vi "Decode Status.vi"(8 "error in (no error)":errorcluster, 10 "Status Line":string) -> (0 "error out":errorcluster, 1 "Checksum OK":bool, 2 "Output":i32)   [LabVIEW 2016]
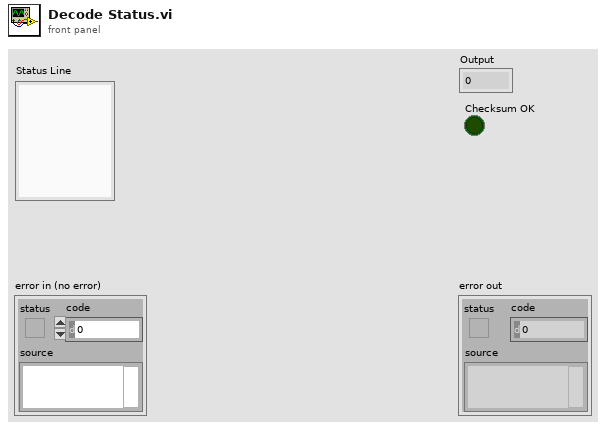
[diagram p1: front panel]
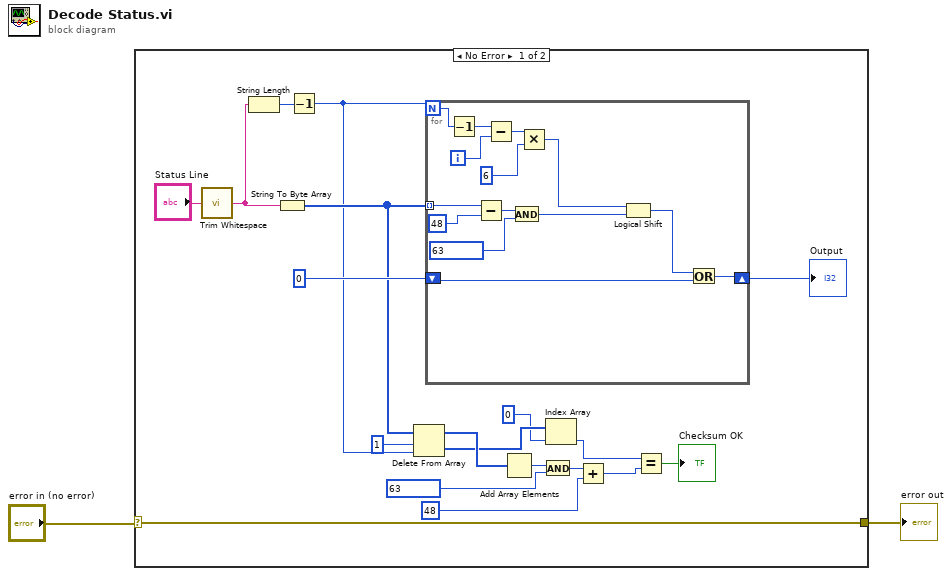
[diagram p0: block diagram]
diagram:
  n1 = case shown="No Error" "error in (no error)" {
    selector: "error in (no error)" -> [w3 w36]
    tunnel: [w3 w36] -> w1
    frame No Error {
      n2 = call <vilib>:"Trim Whitespace.vi"("string"="Status Line") -> ("trimmed string"=w4:string)  [unwired: 1 in]
      n3 = String Length(string=w4) -> (length=w21:i32)
      n4 = String To Byte Array(string=w4) -> (unsigned byte array=w12:u8[])
      n5 = Decrement(x=w21) -> (x-1=w7:i32)
      n6 = Delete From Array(array=w12, length=1, index=w7) -> (deleted portion=w11:u8[], array with subset deleted=w14:u8[])
      n7 = for {
        N: w7 -> [w26]
        tunnel: w12 -> [w22] mode=indexing
        shift-right: [w34] -> w20
        shift-left: 0 -> [w33]
        i -> [w31]
        n8 = Decrement(x=w26) -> (x-1=w25:i32)
        n9 = Subtract(x=w22, y=u8 48) -> (x-y=w28:u8)
        n10 = Subtract(x=w25, y=w31) -> (x-y=w30:i32)
        n11 = And(x=w28, y=u8 63) -> (x .and. y?=w23:u8)
        n12 = Multiply(x=w30, y=6) -> (x*y=w24:i32)
        n13 = Logical Shift(y=w24, x=w23) -> (x << y=w32:u8)
        n14 = Or(x=w32, y=w33) -> (x .or. y?=w34:i32)
      }
      "Output" <- w20
      n15 = Add Array Elements(numeric array=w14) -> (sum=w17:u8)
      n16 = And(x=w17, y=u8 63) -> (x .and. y?=w16:u8)
      n17 = Index Array(array=w11, index=0) -> (element=w9:u8)
      n18 = Add(x=w16, y=u8 48) -> (x+y=w13:u8)
      n19 = Equal?(x=w9, y=w13) -> (x = y?=→"Checksum OK":bool)
    }
    frame Error {
    }
  }
  "error out" <- w1
